vi "Design Filter.vi"(6 "order":i32=7, 7 "Type":T2=enum."Lowpass", 8 "Class":enum16{"Elliptic", "Butterworth"}(ring), 9 "low cutoff freq: fl":dbl=0.125 format="%0.3f", 10 "high cutoff freq: fh":dbl=0.45 format="%0.3f", 11 "sampling freq: fs":dbl=1.0 format="%0.2f") -> (0 "error":i32, 3 "IIR Filter":T1)   [LabVIEW 2020, in "Filter.lvclass"]
uses:
  Filter.lvclass
  Shape.ctl
  <vilib>/Analysis/NI_AALBase.lvlib
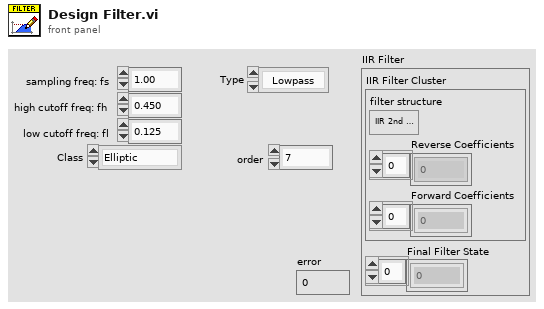
[diagram p1: front panel]
types:
  T1 = cluster{"IIR Filter Cluster":cluster{"filter structure":enum32{"IIR 2nd Order", "IIR 4th Order"}, "Reverse Coefficients":dbl[], "Forward Coefficients":dbl[]}, "Final Filter State":dbl[]}
  T2 = typedef "Filter.lvclass/Shape.ctl" = enum16{"OFF", "Lowpass", "Highpass", "Bandpass", "Bandstop"}
  T3 = cluster{"filter structure":enum32{"IIR 2nd Order", "IIR 4th Order"}, "Reverse Coefficients":dbl[], "Forward Coefficients":dbl[]}
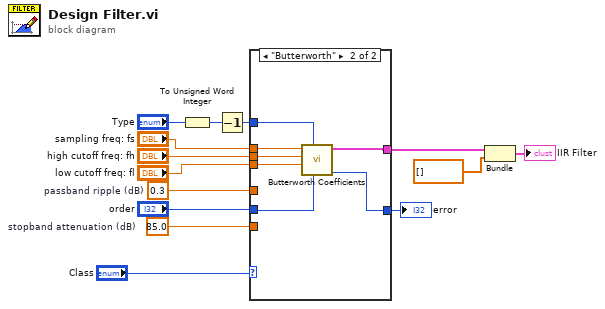
[diagram p0: block diagram]
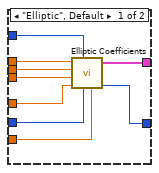
[diagram p2: hidden frame]
diagram:
  w12 = 85.0  # stopband attenuation (dB)
  w14 = 0.3  # passband ripple (dB)
  n1 = To Unsigned Word Integer(number="Type") -> (unsigned 16bit integer=w2:u16)
  n2 = Decrement(x=w2) -> (x-1=w1:u16)
  n3 = case shown="\"Butterworth\"" "Class" {
    tunnel: w14 -> [w23 _]
    tunnel: "order" -> [w22 w26]
    tunnel: w12 -> [w21 _]
    tunnel: w1 -> [w20 w29]
    tunnel: "sampling freq: fs" -> [w19 w30]
    tunnel: "high cutoff freq: fh" -> [w18 w28]
    tunnel: "low cutoff freq: fl" -> [w17 w27]
    tunnel: [w16 w25] -> w7
    tunnel: [w15 w24] -> w3
    frame "Elliptic", Default {
      n4 = call <vilib>:"Elliptic Coefficients.vi"("stopband attenuation (dB)"=w21, "order"=w22, "filter type"=w20, "passband ripple (dB)"=w23, "low cutoff freq: fl"=w17, "high cutoff freq: fh"=w18, "sampling freq: fs"=w19) -> ("error"=w15:i32, "IIR Filter Cluster"=w16:T3)  [unwired: 3 in]
    }
    frame "Butterworth" {
      n5 = call <vilib>:"Butterworth Coefficients.vi"("order"=w26, "filter type"=w29, "low cutoff freq: fl"=w27, "high cutoff freq: fh"=w28, "sampling freq: fs"=w30) -> ("error"=w24:i32, "IIR Filter Cluster"=w25:T3)  [unwired: 5 in]
    }
  }
  "error" <- w3
  n6 = Bundle("IIR Filter Cluster"=w7, "Final Filter State"=dbl[] []) -> (→"IIR Filter":T1)  [unwired: 1 in]
